vi "CustomExample.vi"() -> ()   [LabVIEW 2019, in "MicronGRPCGeneratedServer.lvlib"]
uses:
  MicronGRPCGeneratedServer.lvlib
  4790ee0a-8b3a-4a65-a6ee-7a43fd5db30d.vi
panel:
  out "error out":errorcluster
  in  "Server Address":string="localhost:50051"
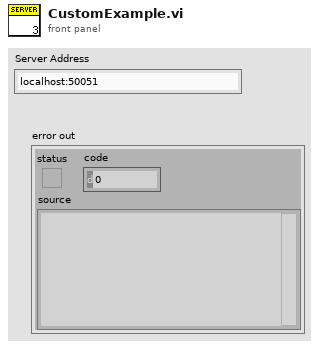
[diagram p1: front panel]
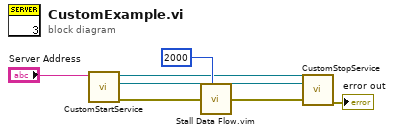
[diagram p0: block diagram]
diagram:
  n1 = call "CustomStartService.vi"("Server Address"="Server Address") -> ("error out"=w7:errorcluster, "Server Stop"=w3:refnum<user-event>, "gRPC Server out"=w2:refnum<class "Servicer.lvclass">)  [unwired: 6 in, 2 out]
  n2 = call "Stall Data Flow.vim"("value in"=w7, "milliseconds to wait"=u32 2000) -> ("value out"=w6:errorcluster)  [unwired: 1 out]
  n3 = call "CustomStopService.vi"("error in (no error)"=w6, "Server Stop"=w3, "gRPC Server"=w2) -> ("error out"=→"error out":errorcluster)  [unwired: 8 in]
